vi "ATF Pump Parameter GUI V1.1.vi"() -> ()   [LabVIEW 2022 SP3]
uses:
  Source code/Globals/Main_global.vi
  Source code/Globals/ATF1_ACQ.vi
panel:
  out "A_NDB":dbl format="%.2f"
  out "A_DB":dbl format="%.2f"
  out "V_NDB":dbl format="%.2f"
  out "V_DB":dbl format="%.2f"
  out "H_NDB":dbl format="%.2f"
  out "H_DB":dbl format="%.2f"
  out "A NDB 2":dbl format="%#.2f"
  out "A DB 2":dbl format="%#.2f"
  out "V_NDB 2":dbl format="%#.2f"
  out "V DB 2":dbl format="%#.2f"
  out "H NDB 2":dbl format="%#.2f"
  out "H DB  2":dbl format="%#.2f"
  out "Speed(RPM)":dbl format="%#.2f"
  out "Torque":dbl format="%#.2f"
  out "PUMP HEAD   =":dbl format="%#.2f"
  out "Speed (RPM)":dbl format="%#.2f"
  out "F_SC_RTD (K)":dbl format="%#.2f"
  out "F-SC-PT(bar)":dbl format="%#.2f"
  out "F_RTD_1013 (K)":dbl format="%#.2f"
  out "F_PT_1013a (bar)":dbl format="%#.2f"
  out "F_RTD_1011 (K)":dbl format="%#.2f"
  out "F_PT_1011a (bar)":dbl format="%#.2f"
  out "F_FM-1010 (g/s)":dbl format="%#.2f"
  out "F_PT_1013b (bar)":dbl format="%#.2f"
  out "F_PT_1011b (bar)":dbl format="%#.2f"
  out "Current (A)":dbl format="%#.2f"
  out "Voltage (V)":dbl format="%#.2f"
  out "D_Dyna_PT (bar)":dbl format="%#.2f"
  out "S_Dyna_PT (bar)":dbl format="%#.2f"
  out "F_PT_9 (bar)":dbl format="%#.2f"
  out "F_PT_8 (bar)":dbl format="%#.2f"
  out "F_PT_5 (bar)":dbl format="%#.2f"
  out "F_PT_6 (bar)":dbl format="%#.2f"
  out "F_PT_7 (bar)":dbl format="%#.2f"
  out "F_PT_4 (bar)":dbl format="%#.2f"
  out "F_PT_1 (bar)":dbl format="%#.2f"
  out "F_PT_2 (bar)":dbl format="%#.2f"
  out "F_PT_3 (bar)":dbl format="%#.2f"
  out "ND B 2 (K)":dbl format="%#.2f"
  out "RTD OUT (K)":dbl format="%#.2f"
  out "ND B 1(K)":dbl format="%#.2f"
  out "DE Bearing T (C))":dbl format="%#.2f"
  out "Motor Outer\n body Temp(C)":dbl format="%#.2f"
  out "NDE Bearing T (C)":dbl format="%#.2f"
  out "P_TC5 (k)":dbl format="%#.2f"
  out "P_TC4 (k)":dbl format="%#.2f"
  out "P_TC3 (K)":dbl format="%#.2f"
  out "P_RTD (k)":dbl format="%#.2f"
  out "P_TC2 (k)":dbl format="%#.2f"
  out "P_TC1 (k)":dbl format="%#.2f"
  # "ATF Rig Parameters GUI V1.0"
  # "THERMAL DATA"
  # "PRESSURE DATA"
  # "CRITICAL DATA"
  # "VIBRATION DATA"
  # "MOTOR"
  # "NDB"
  # "DB"
  # "g"
  # "g"
  # "H"
  # "g"
  # "V"
  # "g"
  # "g"
  # "g"
  # "A"
  # "PUMP"
  # "BEARING"
  # "PUMP"
  # "g"
  # "H"
  # "g"
  # "g"
  # "V"
  # "g"
  # "g"
  # "A"
  # "g"
  # "TORQUE METER"
  # "DRIVE PARAMETERS"
  # "F_S_Uol_PT"
  # "F_S_Dol_PT"
  # "F_SC_PT"
  # "F_SF_PT"
  # "F_V_PT1"
  # "F_V_PT2"
  # "F_V_PT3"
  # "F_V_PT4"
  # "F_D_PT"
  # "MOTOR"
  # "PUMP"
  # "Version:V0.1"
  # "Release Date:17/10/2024"
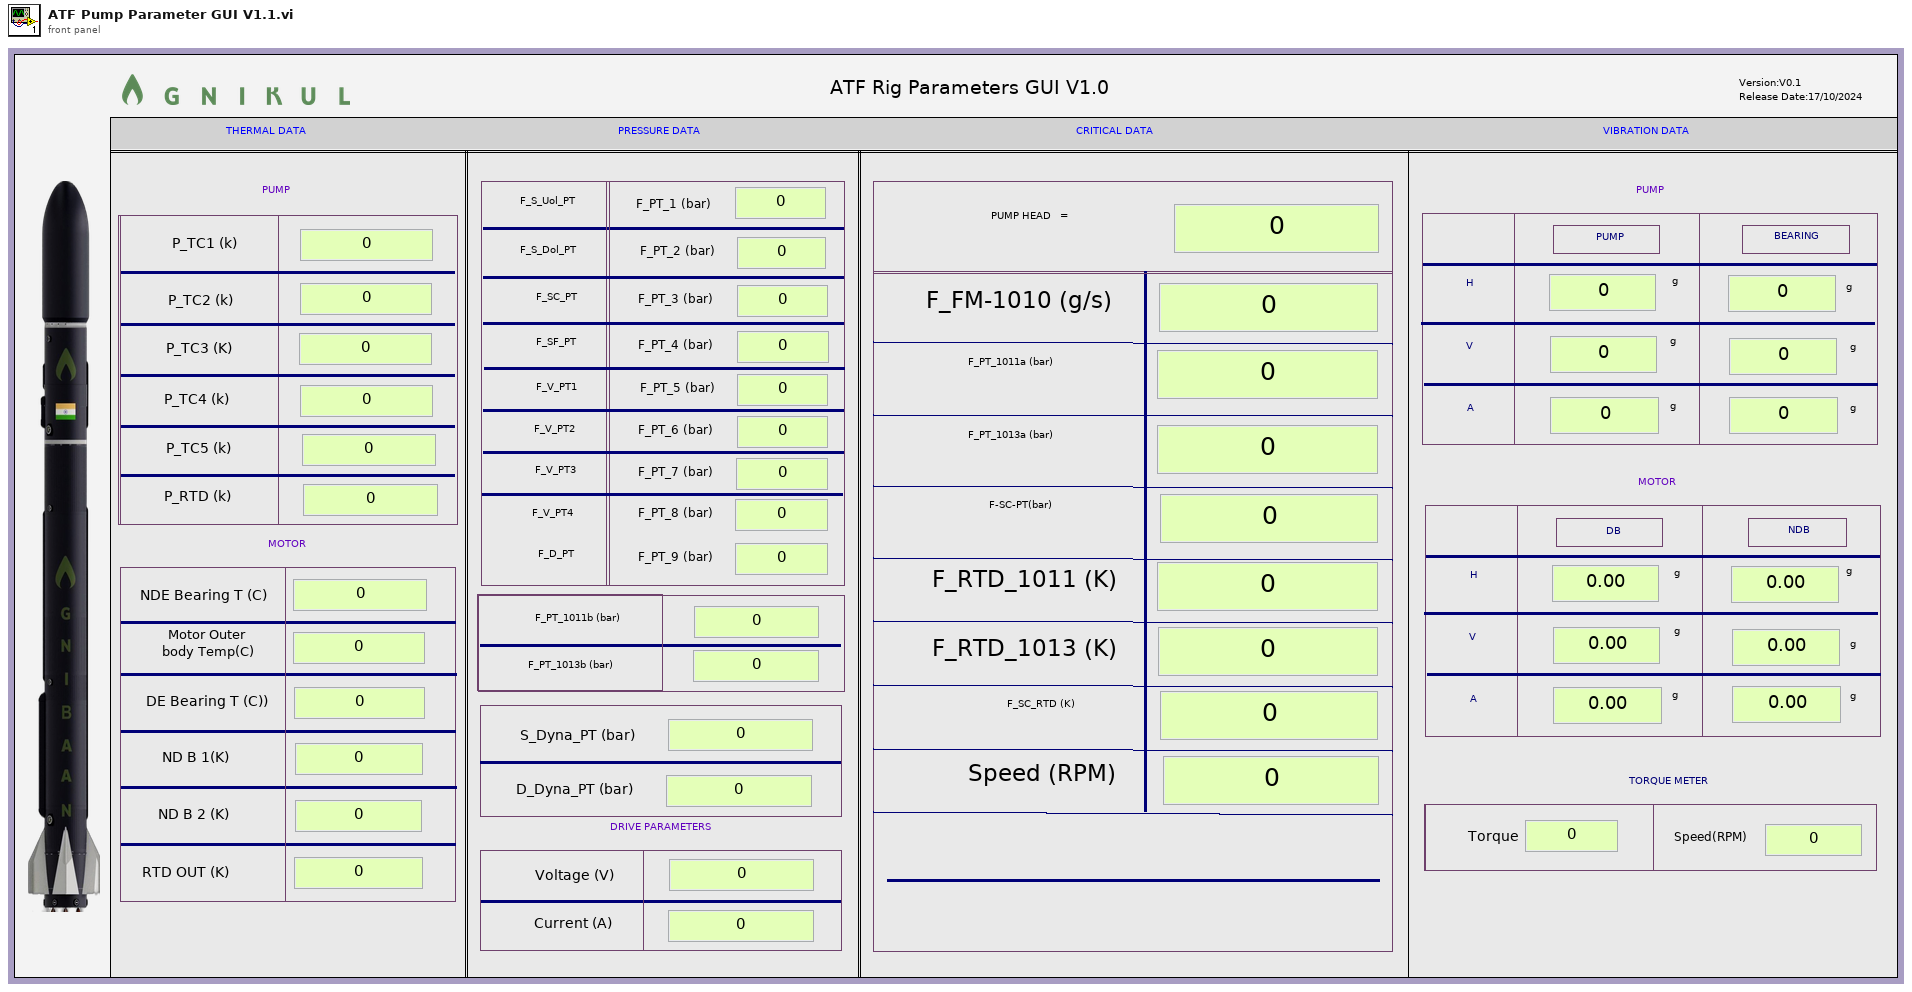
[diagram p1: front panel]
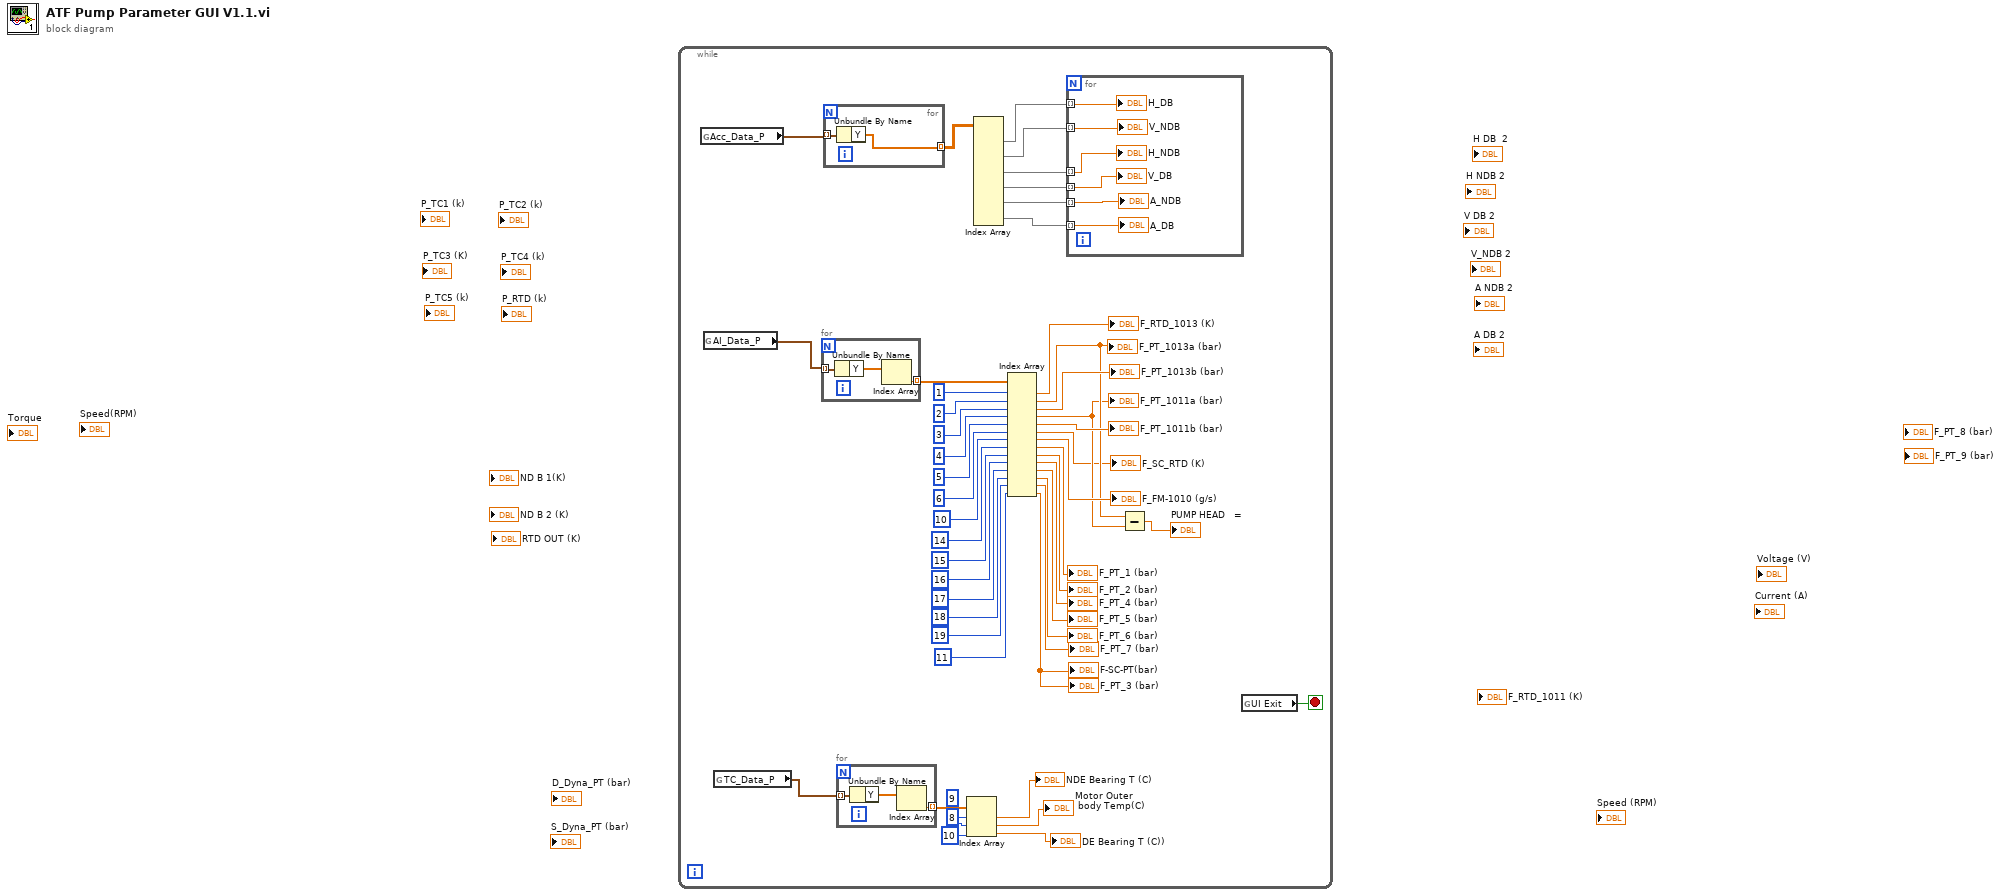
[diagram p0: block diagram]
diagram:
  n1 = while {
    stop <- w33 stop-if-true
    n2 = global read "ATF1_ACQ.vi" "Acc_Data_P"() -> (w25:waveform(dbl)[])
    n3 = global read "ATF1_ACQ.vi" "AI_Data_P"() -> (w24:waveform(dbl)[])
    n4 = global read "ATF1_ACQ.vi" "TC_Data_P"() -> (w8:waveform(dbl)[])
    n5 = for {
      tunnel: w24 -> [w61] mode=indexing
      tunnel: [w60] -> w41 mode=indexing
      n6 = Unbundle By Name(w61) -> ("Y"=w62:dbl[])
      n7 = Index Array(array=w62) -> (element=w60:dbl)  [unwired: 1 in]
    }
    n8 = for {
      tunnel: w25 -> [w58] mode=indexing
      tunnel: [w59] -> w32 mode=indexing
      n9 = Unbundle By Name(w58) -> ("Y"=w59:dbl[])
    }
    n10 = for {
      tunnel: [w57] -> w7 mode=indexing
      tunnel: w8 -> [w56] mode=indexing
      n11 = Unbundle By Name(w56) -> ("Y"=w55:dbl[])
      n12 = Index Array(array=w55) -> (element=w57:dbl)  [unwired: 1 in]
    }
    n13 = Index Array(array=w7, index #1=8 ("index"), index #2=9 ("index"), index #3=10 ("index")) -> (element #1=→"NDE Bearing T (C)":dbl, element #2=→"Motor Outer\n body Temp(C)":dbl, element #3=→"DE Bearing T (C))":dbl)
    n14 = Index Array(array=w32) -> (element #1=w31:dbl[], element #2=w30:dbl[], element #3=w29:dbl[], element #4=w28:dbl[], element #5=w27:dbl[], element #6=w26:dbl[])  [unwired: 12 in]
    n15 = Index Array(array=w41, index #1=1 ("index"), index #2=2 ("index"), index #3=3 ("index"), index #4=4 ("index"), index #5=5 ("index"), index #6=6 ("index"), index #7=10 ("index"), index #8=14 ("index"), index #9=15 ("index"), index #10=16 ("index"), index #11=17 ("index"), index #12=18 ("index"), index #13=19 ("index"), index #14=11 ("index")) -> (element #1=→"F_RTD_1013 (K)":dbl, element #2=w35:dbl, element #3=→"F_PT_1013b (bar)":dbl, element #4=w34:dbl, element #5=→"F_PT_1011b (bar)":dbl, element #6=→"F_SC_RTD (K)":dbl, element #7=→"F_FM-1010 (g/s)":dbl, element #8=→"F_PT_1 (bar)":dbl, element #9=→"F_PT_2 (bar)":dbl, element #10=→"F_PT_4 (bar)":dbl, element #11=→"F_PT_5 (bar)":dbl, element #12=→"F_PT_6 (bar)":dbl, element #13=→"F_PT_7 (bar)":dbl, element #14=→"F_PT_3 (bar)" →"F-SC-PT(bar)":dbl)
    "F_PT_1013a (bar)" <- w35
    "F_PT_1011a (bar)" <- w34
    n16 = for {
      tunnel: w31 -> [w54] mode=indexing
      tunnel: w30 -> [w53] mode=indexing
      tunnel: w29 -> [w52] mode=indexing
      tunnel: w28 -> [w51] mode=indexing
      tunnel: w27 -> [w50] mode=indexing
      tunnel: w26 -> [w49] mode=indexing
      "H_DB" <- w54
      "H_NDB" <- w52
      "V_DB" <- w51
      "V_NDB" <- w53
      "A_DB" <- w49
      "A_NDB" <- w50
    }
    n17 = Subtract(x=w35, y=w34) -> (x-y=→"PUMP HEAD   =":dbl)
    n18 = global read "Main_global.vi" "UI Exit"() -> (w33:bool)
  }
